vi "noise removal.vi"(8 "after14":dbl, 9 "before14":dbl, 10 "y":dbl, 11 "x":dbl) -> (0 "sdy":dbl format="%0.2f", 1 "sdx":dbl format="%0.2f", 2 "newy":dbl format="%0.2f", 3 "newx":dbl format="%0.2f")   [LabVIEW 2018]
uses:
  <vilib>/Analysis/baseanly.llb/Mean (DBL).vi
  <vilib>/Analysis/NI_AALBase.lvlib
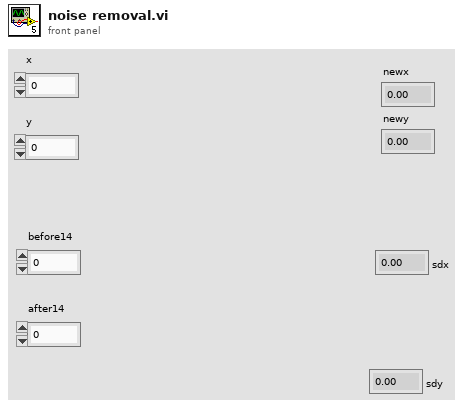
[diagram p1: front panel]
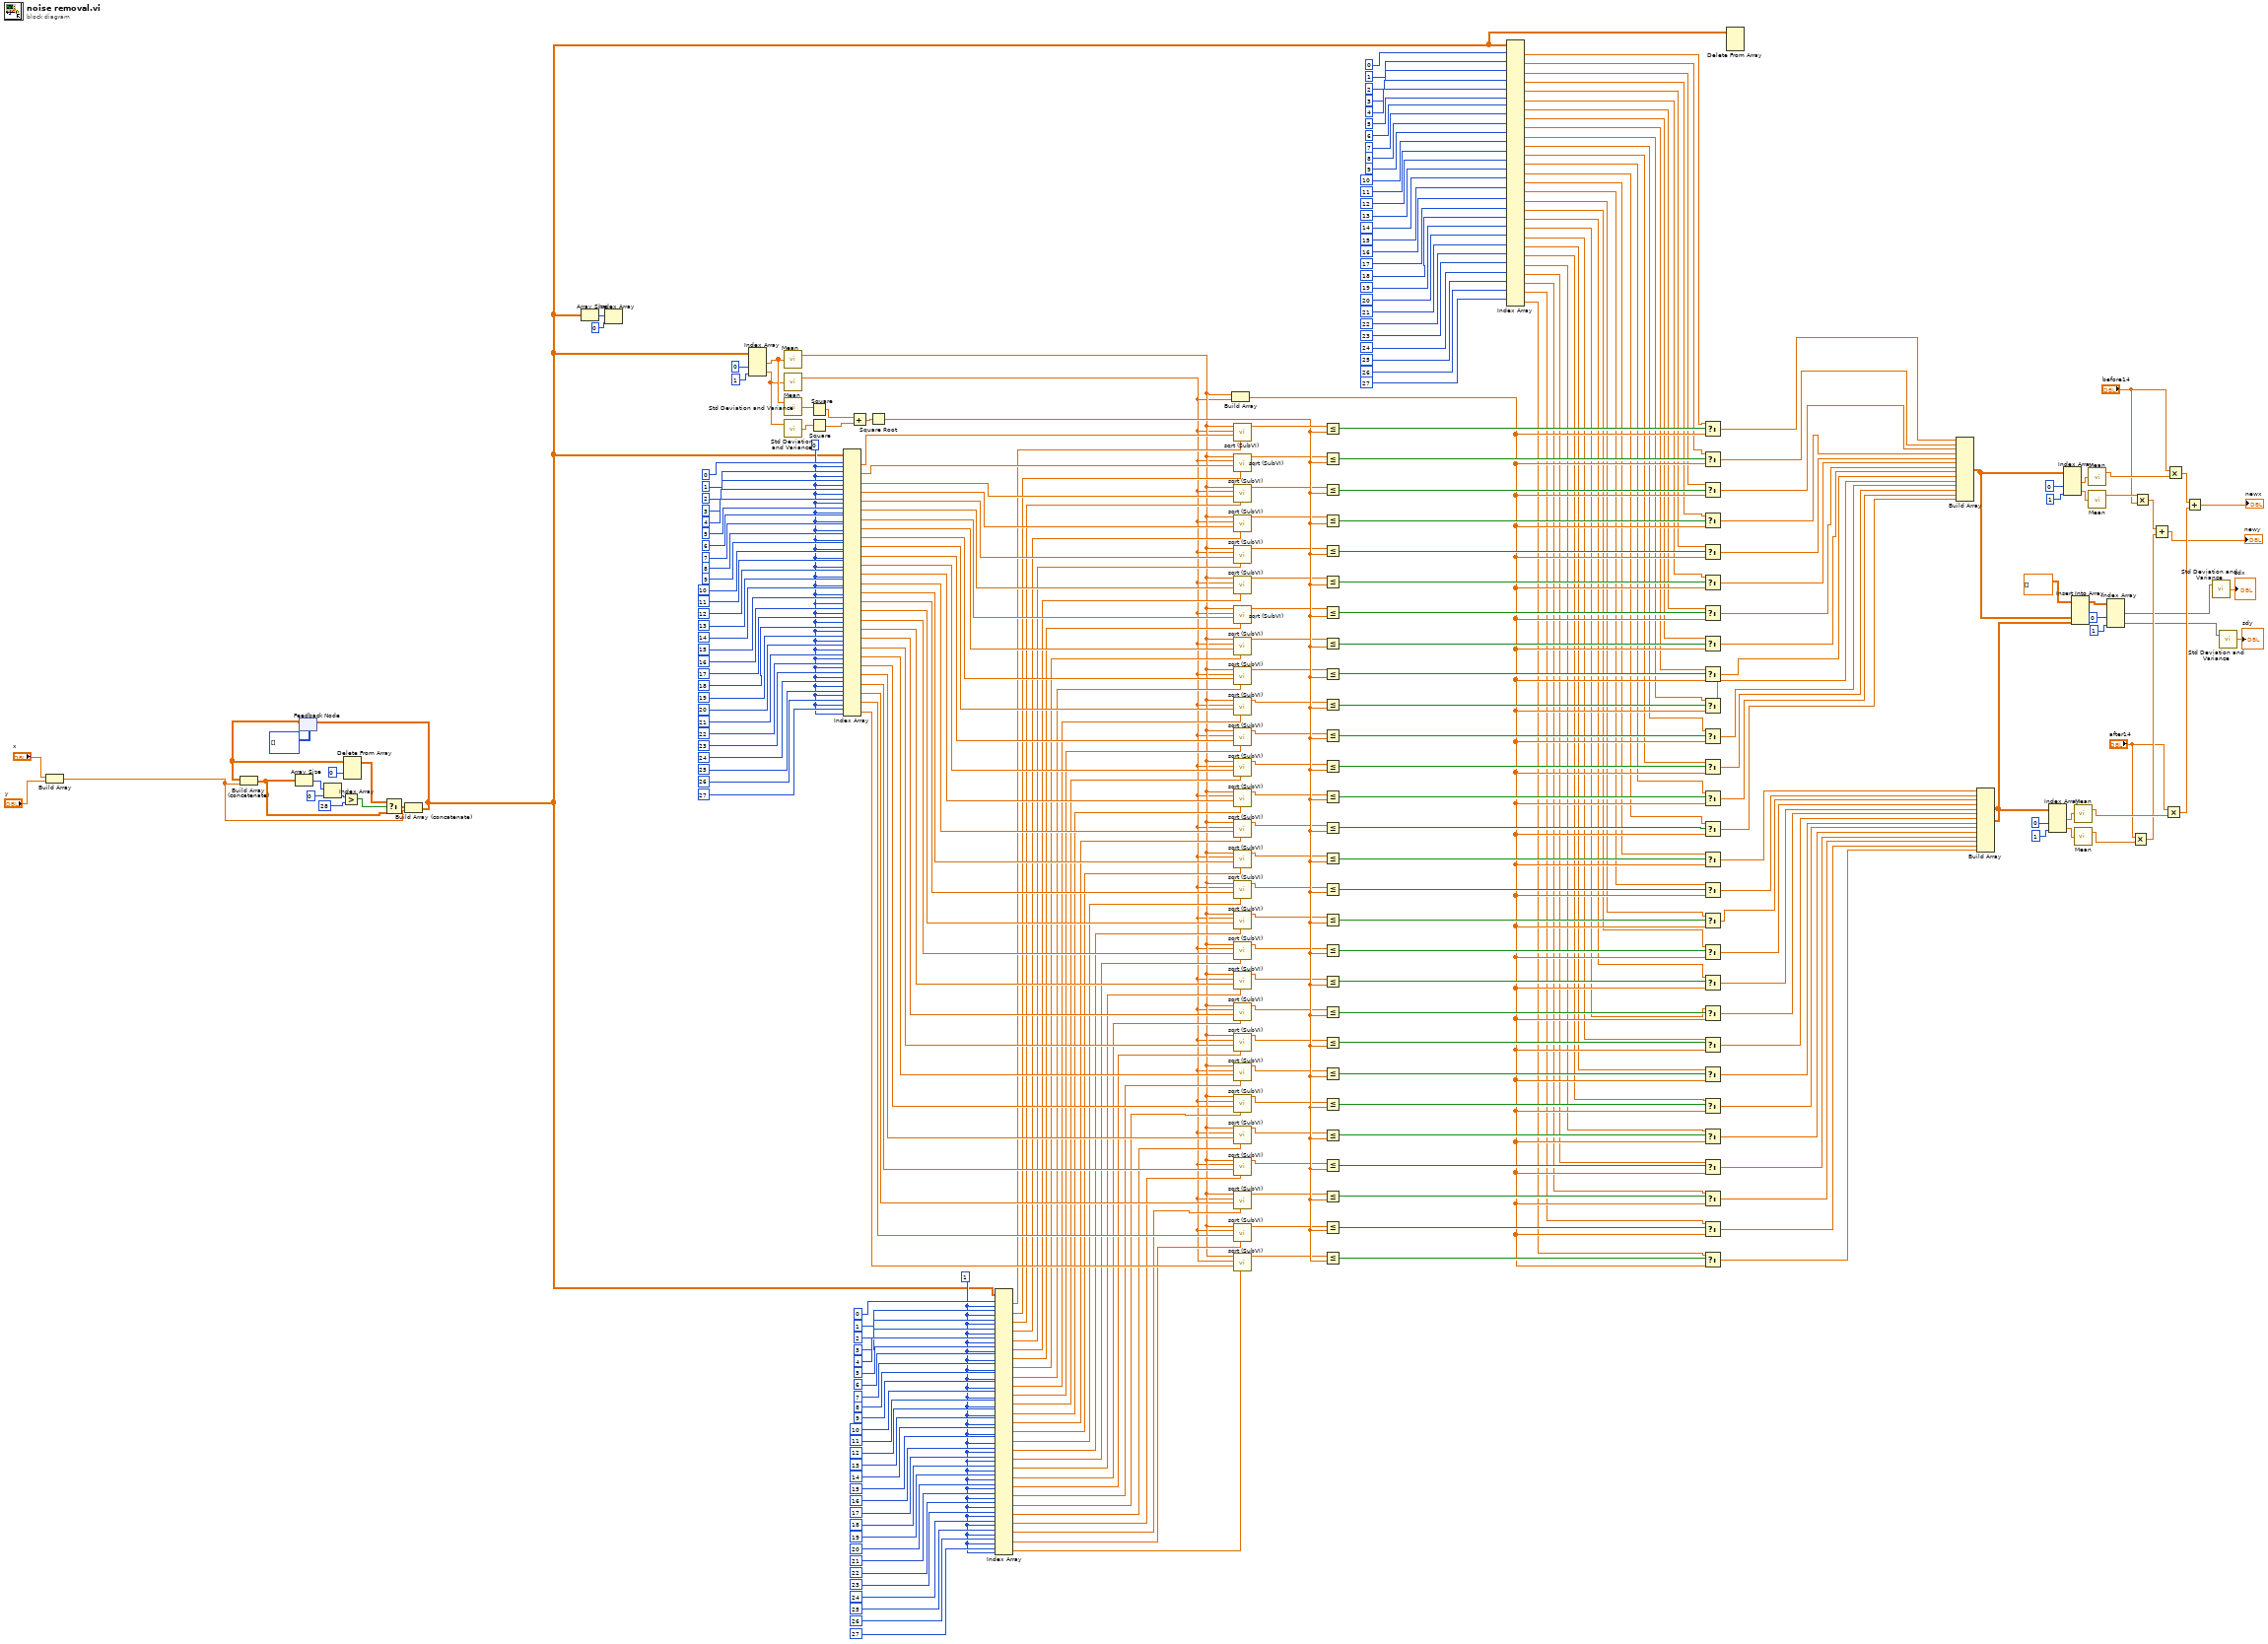
[diagram p0: block diagram]
diagram:
  w239 = 1
  w272 = 0
  n1 = Build Array("x", "y") -> (w314:dbl[])
  n2 = feedback #1(i32[][] []) -> (w299:dbl[][])
  n3 = Build Array (concatenate)(w299, w314) -> (w300:dbl[][])
  n4 = Array Size(array=w300) -> (size(s)=w291:i32[])
  n5 = Index Array(array=w291, index=0) -> (element=w293:i32)
  n6 = Greater?(x=w293, y=28) -> (0:w295:bool)
  n7 = Delete From Array(array=w299, index (row)=0) -> (array with subset deleted=w296:dbl[][])  [unwired: 2 in, 1 out]
  n8 = Select(t=w296, s=w295, f=w300) -> (s? t:f=w313:dbl[][])
  n9 = Build Array (concatenate)(w313, w314) -> (w89:dbl[][])
  n10 = feedback-in #1(w89) -> ()
  n11 = Array Size(array=w89) -> (size(s)=w311:i32[])
  n12 = Index Array(array=w311, index=0) -> ()  [unwired: 1 out]
  n13 = Index Array(array=w89, index (col) #1=0, index (col) #2=1) -> (element #1=w269:dbl[], element #2=w268:dbl[])  [unwired: 2 in]
  n14 = call-poly <vilib>:"Mean.vi"("X"=w269) -> ("mean"=w120:dbl)  [unwired: 1 out]
  n15 = call-poly <vilib>:"Mean.vi"("X"=w268) -> ("mean"=w119:dbl)  [unwired: 1 out]
  n16 = call <vilib>:"Std Deviation and Variance.vi"("X"=w268) -> ("standard deviation"=w234:dbl)  [unwired: 1 in, 2 out]
  n17 = call <vilib>:"Std Deviation and Variance.vi"("X"=w269) -> ("standard deviation"=w235:dbl)  [unwired: 1 in, 2 out]
  n18 = Square(x=w235) -> (x^2=w238:dbl)
  n19 = Square(x=w234) -> (x^2=w237:dbl)
  n20 = Index Array(array=w89, index (row) #1=0, index (col) #1=w272, index (row) #2=1, index (col) #2=w272, index (row) #3=2, index (col) #3=w272, index (row) #4=3, index (col) #4=w272, index (row) #5=4, index (col) #5=w272, index (row) #6=5, index (col) #6=w272, index (row) #7=6, index (col) #7=w272, index (row) #8=7, index (col) #8=w272, index (row) #9=8, index (col) #9=w272, index (row) #10=9, index (col) #10=w272, index (row) #11=10, index (col) #11=w272, index (row) #12=11, index (col) #12=w272, index (row) #13=12, index (col) #13=w272, index (row) #14=13, index (col) #14=w272, index (row) #15=14, index (col) #15=w272, index (row) #16=15, index (col) #16=w272, index (row) #17=16, index (col) #17=w272, index (row) #18=17, index (col) #18=w272, index (row) #19=18, index (col) #19=w272, index (row) #20=19, index (col) #20=w272, index (row) #21=20, index (col) #21=w272, index (row) #22=21, index (col) #22=w272, index (row) #23=22, index (col) #23=w272, index (row) #24=23, index (col) #24=w272, index (row) #25=24, index (col) #25=w272, index (row) #26=25, index (col) #26=w272, index (row) #27=26, index (col) #27=w272, index (row) #28=27, index (col) #28=w272) -> (element #1=w233:dbl, element #2=w232:dbl, element #3=w231:dbl, element #4=w230:dbl, element #5=w229:dbl, element #6=w228:dbl, element #7=w227:dbl, element #8=w226:dbl, element #9=w225:dbl, element #10=w224:dbl, element #11=w223:dbl, element #12=w222:dbl, element #13=w221:dbl, element #14=w220:dbl, element #15=w219:dbl, element #16=w218:dbl, element #17=w217:dbl, element #18=w216:dbl, element #19=w215:dbl, element #20=w214:dbl, element #21=w213:dbl, element #22=w212:dbl, element #23=w211:dbl, element #24=w210:dbl, element #25=w209:dbl, element #26=w208:dbl, element #27=w207:dbl, element #28=w206:dbl)
  n21 = Add(x=w238, y=w237) -> (x+y=w236:dbl)
  n22 = Square Root(x=w236) -> (sqrt(x)=w176:dbl)
  n23 = Index Array(array=w89, index (row) #1=0, index (col) #1=w239, index (row) #2=1, index (col) #2=w239, index (row) #3=2, index (col) #3=w239, index (row) #4=3, index (col) #4=w239, index (row) #5=4, index (col) #5=w239, index (row) #6=5, index (col) #6=w239, index (row) #7=6, index (col) #7=w239, index (row) #8=7, index (col) #8=w239, index (row) #9=8, index (col) #9=w239, index (row) #10=9, index (col) #10=w239, index (row) #11=10, index (col) #11=w239, index (row) #12=11, index (col) #12=w239, index (row) #13=12, index (col) #13=w239, index (row) #14=13, index (col) #14=w239, index (row) #15=14, index (col) #15=w239, index (row) #16=15, index (col) #16=w239, index (row) #17=16, index (col) #17=w239, index (row) #18=17, index (col) #18=w239, index (row) #19=18, index (col) #19=w239, index (row) #20=19, index (col) #20=w239, index (row) #21=20, index (col) #21=w239, index (row) #22=21, index (col) #22=w239, index (row) #23=22, index (col) #23=w239, index (row) #24=23, index (col) #24=w239, index (row) #25=24, index (col) #25=w239, index (row) #26=25, index (col) #26=w239, index (row) #27=26, index (col) #27=w239, index (row) #28=27, index (col) #28=w239) -> (element #1=w205:dbl, element #2=w204:dbl, element #3=w203:dbl, element #4=w202:dbl, element #5=w201:dbl, element #6=w200:dbl, element #7=w199:dbl, element #8=w198:dbl, element #9=w197:dbl, element #10=w196:dbl, element #11=w195:dbl, element #12=w194:dbl, element #13=w193:dbl, element #14=w192:dbl, element #15=w191:dbl, element #16=w190:dbl, element #17=w189:dbl, element #18=w188:dbl, element #19=w187:dbl, element #20=w186:dbl, element #21=w185:dbl, element #22=w184:dbl, element #23=w183:dbl, element #24=w182:dbl, element #25=w181:dbl, element #26=w180:dbl, element #27=w179:dbl, element #28=w178:dbl)
  n24 = Build Array(w120, w119) -> (w90:dbl[])
  n25 = call "sqrt (SubVI).vi"("y"=w205, "x"=w233, "ym"=w119, "xm"=w120) -> ("sq"=w177:dbl)  [unwired: 7 in]
  n26 = call "sqrt (SubVI).vi"("y"=w204, "x"=w232, "ym"=w119, "xm"=w120) -> ("sq"=w175:dbl)  [unwired: 7 in]
  n27 = call "sqrt (SubVI).vi"("y"=w203, "x"=w231, "ym"=w119, "xm"=w120) -> ("sq"=w174:dbl)  [unwired: 7 in]
  n28 = call "sqrt (SubVI).vi"("y"=w202, "x"=w230, "ym"=w119, "xm"=w120) -> ("sq"=w173:dbl)  [unwired: 7 in]
  n29 = call "sqrt (SubVI).vi"("y"=w201, "x"=w229, "ym"=w119, "xm"=w120) -> ("sq"=w172:dbl)  [unwired: 7 in]
  n30 = call "sqrt (SubVI).vi"("y"=w200, "x"=w228, "ym"=w119, "xm"=w120) -> ("sq"=w171:dbl)  [unwired: 7 in]
  n31 = call "sqrt (SubVI).vi"("y"=w199, "x"=w227, "ym"=w119, "xm"=w120) -> ("sq"=w170:dbl)  [unwired: 7 in]
  n32 = call "sqrt (SubVI).vi"("y"=w198, "x"=w226, "ym"=w119, "xm"=w120) -> ("sq"=w169:dbl)  [unwired: 7 in]
  n33 = call "sqrt (SubVI).vi"("y"=w197, "x"=w225, "ym"=w119, "xm"=w120) -> ("sq"=w168:dbl)  [unwired: 7 in]
  n34 = call "sqrt (SubVI).vi"("y"=w196, "x"=w224, "ym"=w119, "xm"=w120) -> ("sq"=w167:dbl)  [unwired: 7 in]
  n35 = call "sqrt (SubVI).vi"("y"=w195, "x"=w223, "ym"=w119, "xm"=w120) -> ("sq"=w166:dbl)  [unwired: 7 in]
  n36 = call "sqrt (SubVI).vi"("y"=w194, "x"=w222, "ym"=w119, "xm"=w120) -> ("sq"=w165:dbl)  [unwired: 7 in]
  n37 = call "sqrt (SubVI).vi"("y"=w193, "x"=w221, "ym"=w119, "xm"=w120) -> ("sq"=w164:dbl)  [unwired: 7 in]
  n38 = call "sqrt (SubVI).vi"("y"=w192, "x"=w220, "ym"=w119, "xm"=w120) -> ("sq"=w163:dbl)  [unwired: 7 in]
  n39 = call "sqrt (SubVI).vi"("y"=w191, "x"=w219, "ym"=w119, "xm"=w120) -> ("sq"=w162:dbl)  [unwired: 7 in]
  n40 = call "sqrt (SubVI).vi"("y"=w190, "x"=w218, "ym"=w119, "xm"=w120) -> ("sq"=w161:dbl)  [unwired: 7 in]
  n41 = call "sqrt (SubVI).vi"("y"=w189, "x"=w217, "ym"=w119, "xm"=w120) -> ("sq"=w160:dbl)  [unwired: 7 in]
  n42 = call "sqrt (SubVI).vi"("y"=w188, "x"=w216, "ym"=w119, "xm"=w120) -> ("sq"=w159:dbl)  [unwired: 7 in]
  n43 = call "sqrt (SubVI).vi"("y"=w187, "x"=w215, "ym"=w119, "xm"=w120) -> ("sq"=w158:dbl)  [unwired: 7 in]
  n44 = call "sqrt (SubVI).vi"("y"=w186, "x"=w214, "ym"=w119, "xm"=w120) -> ("sq"=w157:dbl)  [unwired: 7 in]
  n45 = call "sqrt (SubVI).vi"("y"=w185, "x"=w213, "ym"=w119, "xm"=w120) -> ("sq"=w156:dbl)  [unwired: 7 in]
  n46 = call "sqrt (SubVI).vi"("y"=w184, "x"=w212, "ym"=w119, "xm"=w120) -> ("sq"=w155:dbl)  [unwired: 7 in]
  n47 = call "sqrt (SubVI).vi"("y"=w183, "x"=w211, "ym"=w119, "xm"=w120) -> ("sq"=w154:dbl)  [unwired: 7 in]
  n48 = call "sqrt (SubVI).vi"("y"=w182, "x"=w210, "ym"=w119, "xm"=w120) -> ("sq"=w153:dbl)  [unwired: 7 in]
  n49 = call "sqrt (SubVI).vi"("y"=w181, "x"=w209, "ym"=w119, "xm"=w120) -> ("sq"=w152:dbl)  [unwired: 7 in]
  n50 = call "sqrt (SubVI).vi"("y"=w180, "x"=w208, "ym"=w119, "xm"=w120) -> ("sq"=w151:dbl)  [unwired: 7 in]
  n51 = call "sqrt (SubVI).vi"("y"=w179, "x"=w207, "ym"=w119, "xm"=w120) -> ("sq"=w150:dbl)  [unwired: 7 in]
  n52 = call "sqrt (SubVI).vi"("y"=w178, "x"=w206, "ym"=w119, "xm"=w120) -> ("sq"=w149:dbl)  [unwired: 7 in]
  n53 = Less Or Equal?(x=w177, y=w176) -> (x <= y?=w118:bool)
  n54 = Less Or Equal?(x=w175, y=w176) -> (x <= y?=w117:bool)
  n55 = Less Or Equal?(x=w174, y=w176) -> (x <= y?=w116:bool)
  n56 = Less Or Equal?(x=w173, y=w176) -> (x <= y?=w115:bool)
  n57 = Less Or Equal?(x=w172, y=w176) -> (x <= y?=w114:bool)
  n58 = Less Or Equal?(x=w171, y=w176) -> (x <= y?=w113:bool)
  n59 = Less Or Equal?(x=w170, y=w176) -> (x <= y?=w112:bool)
  n60 = Less Or Equal?(x=w169, y=w176) -> (x <= y?=w111:bool)
  n61 = Less Or Equal?(x=w168, y=w176) -> (x <= y?=w110:bool)
  n62 = Less Or Equal?(x=w167, y=w176) -> (x <= y?=w109:bool)
  n63 = Less Or Equal?(x=w166, y=w176) -> (x <= y?=w108:bool)
  n64 = Less Or Equal?(x=w165, y=w176) -> (x <= y?=w107:bool)
  n65 = Less Or Equal?(x=w164, y=w176) -> (x <= y?=w106:bool)
  n66 = Less Or Equal?(x=w163, y=w176) -> (x <= y?=w105:bool)
  n67 = Less Or Equal?(x=w162, y=w176) -> (x <= y?=w104:bool)
  n68 = Less Or Equal?(x=w161, y=w176) -> (x <= y?=w103:bool)
  n69 = Less Or Equal?(x=w160, y=w176) -> (x <= y?=w102:bool)
  n70 = Less Or Equal?(x=w159, y=w176) -> (x <= y?=w101:bool)
  n71 = Less Or Equal?(x=w158, y=w176) -> (x <= y?=w100:bool)
  n72 = Less Or Equal?(x=w157, y=w176) -> (x <= y?=w99:bool)
  n73 = Less Or Equal?(x=w156, y=w176) -> (x <= y?=w98:bool)
  n74 = Less Or Equal?(x=w155, y=w176) -> (x <= y?=w97:bool)
  n75 = Less Or Equal?(x=w154, y=w176) -> (x <= y?=w96:bool)
  n76 = Less Or Equal?(x=w153, y=w176) -> (x <= y?=w95:bool)
  n77 = Less Or Equal?(x=w152, y=w176) -> (x <= y?=w94:bool)
  n78 = Less Or Equal?(x=w151, y=w176) -> (x <= y?=w93:bool)
  n79 = Less Or Equal?(x=w150, y=w176) -> (x <= y?=w92:bool)
  n80 = Less Or Equal?(x=w149, y=w176) -> (x <= y?=w91:bool)
  n81 = Index Array(array=w89, index (row) #1=0, index (row) #2=1, index (row) #3=2, index (row) #4=3, index (row) #5=4, index (row) #6=5, index (row) #7=6, index (row) #8=7, index (row) #9=8, index (row) #10=9, index (row) #11=10, index (row) #12=11, index (row) #13=12, index (row) #14=13, index (row) #15=14, index (row) #16=15, index (row) #17=16, index (row) #18=17, index (row) #19=18, index (row) #20=19, index (row) #21=20, index (row) #22=21, index (row) #23=22, index (row) #24=23, index (row) #25=24, index (row) #26=25, index (row) #27=26, index (row) #28=27) -> (element #1=w88:dbl[], element #2=w87:dbl[], element #3=w86:dbl[], element #4=w85:dbl[], element #5=w84:dbl[], element #6=w83:dbl[], element #7=w82:dbl[], element #8=w81:dbl[], element #9=w80:dbl[], element #10=w79:dbl[], element #11=w78:dbl[], element #12=w77:dbl[], element #13=w76:dbl[], element #14=w75:dbl[], element #15=w74:dbl[], element #16=w73:dbl[], element #17=w72:dbl[], element #18=w71:dbl[], element #19=w70:dbl[], element #20=w69:dbl[], element #21=w68:dbl[], element #22=w67:dbl[], element #23=w66:dbl[], element #24=w65:dbl[], element #25=w64:dbl[], element #26=w63:dbl[], element #27=w62:dbl[], element #28=w61:dbl[])  [unwired: 28 in]
  n82 = Select(t=w88, s=w118, f=w90) -> (s? t:f=w56:dbl[])
  n83 = Select(t=w87, s=w117, f=w90) -> (s? t:f=w55:dbl[])
  n84 = Select(t=w86, s=w116, f=w90) -> (s? t:f=w54:dbl[])
  n85 = Select(t=w85, s=w115, f=w90) -> (s? t:f=w53:dbl[])
  n86 = Select(t=w84, s=w114, f=w90) -> (s? t:f=w52:dbl[])
  n87 = Select(t=w83, s=w113, f=w90) -> (s? t:f=w51:dbl[])
  n88 = Select(t=w82, s=w112, f=w90) -> (s? t:f=w50:dbl[])
  n89 = Select(t=w81, s=w111, f=w90) -> (s? t:f=w49:dbl[])
  n90 = Select(t=w80, s=w110, f=w90) -> (s? t:f=w48:dbl[])
  n91 = Select(t=w79, s=w109, f=w90) -> (s? t:f=w47:dbl[])
  n92 = Select(t=w78, s=w108, f=w90) -> (s? t:f=w46:dbl[])
  n93 = Select(t=w77, s=w107, f=w90) -> (s? t:f=w45:dbl[])
  n94 = Select(t=w76, s=w106, f=w90) -> (s? t:f=w44:dbl[])
  n95 = Select(t=w75, s=w105, f=w90) -> (s? t:f=w43:dbl[])
  n96 = Select(t=w74, s=w104, f=w90) -> (s? t:f=w28:dbl[])
  n97 = Select(t=w73, s=w103, f=w90) -> (s? t:f=w29:dbl[])
  n98 = Select(t=w72, s=w102, f=w90) -> (s? t:f=w30:dbl[])
  n99 = Select(t=w71, s=w101, f=w90) -> (s? t:f=w31:dbl[])
  n100 = Select(t=w70, s=w100, f=w90) -> (s? t:f=w32:dbl[])
  n101 = Select(t=w69, s=w99, f=w90) -> (s? t:f=w33:dbl[])
  n102 = Select(t=w68, s=w98, f=w90) -> (s? t:f=w34:dbl[])
  n103 = Select(t=w67, s=w97, f=w90) -> (s? t:f=w35:dbl[])
  n104 = Select(t=w66, s=w96, f=w90) -> (s? t:f=w36:dbl[])
  n105 = Select(t=w65, s=w95, f=w90) -> (s? t:f=w37:dbl[])
  n106 = Select(t=w64, s=w94, f=w90) -> (s? t:f=w38:dbl[])
  n107 = Select(t=w63, s=w93, f=w90) -> (s? t:f=w39:dbl[])
  n108 = Select(t=w62, s=w92, f=w90) -> (s? t:f=w40:dbl[])
  n109 = Select(t=w61, s=w91, f=w90) -> (s? t:f=w41:dbl[])
  n110 = Delete From Array(array=w89) -> ()  [unwired: 3 in, 2 out]
  n111 = Build Array(w56, w55, w54, w53, w52, w51, w50, w49, w48, w47, w46, w45, w44, w43) -> (w11:dbl[][])
  n112 = Build Array(w28, w29, w30, w31, w32, w33, w34, w35, w36, w37, w38, w39, w40, w41) -> (w10:dbl[][])
  n113 = Index Array(array=w10, index (col) #1=0, index (col) #2=1) -> (element #1=w24:dbl[], element #2=w23:dbl[])  [unwired: 2 in]
  n114 = Index Array(array=w11, index (col) #1=0, index (col) #2=1) -> (element #1=w58:dbl[], element #2=w57:dbl[])  [unwired: 2 in]
  n115 = Insert Into Array(array=dbl[][] [], new element #1=w11, new element #2=w10) -> (w7:dbl[][])  [unwired: 2 in]
  n116 = call-poly <vilib>:"Mean.vi"("X"=w24) -> ("mean"=w21:dbl)  [unwired: 1 out]
  n117 = call-poly <vilib>:"Mean.vi"("X"=w23) -> ("mean"=w15:dbl)  [unwired: 1 out]
  n118 = call-poly <vilib>:"Mean.vi"("X"=w58) -> ("mean"=w22:dbl)  [unwired: 1 out]
  n119 = call-poly <vilib>:"Mean.vi"("X"=w57) -> ("mean"=w18:dbl)  [unwired: 1 out]
  n120 = Index Array(array=w7, index (col) #1=0, index (col) #2=1) -> (element #1=w6:dbl[], element #2=w5:dbl[])  [unwired: 2 in]
  n121 = Multiply(x="after14", y=w15) -> (x*y=w19:dbl)
  n122 = Multiply(x=w18, y="before14") -> (x*y=w20:dbl)
  n123 = Add(x=w20, y=w19) -> (x+y=→"newy":dbl)
  n124 = Multiply(x="after14", y=w21) -> (x*y=w27:dbl)
  n125 = Multiply(x="before14", y=w22) -> (x*y=w42:dbl)
  n126 = Add(x=w42, y=w27) -> (x+y=→"newx":dbl)
  n127 = call <vilib>:"Std Deviation and Variance.vi"("X"=w6) -> ("standard deviation"=→"sdx":dbl)  [unwired: 1 in, 2 out]
  n128 = call <vilib>:"Std Deviation and Variance.vi"("X"=w5) -> ("standard deviation"=→"sdy":dbl)  [unwired: 1 in, 2 out]
